vi "Is Close Delimiter.vi"(8 "Error In":errorcluster, 11 "Lexer In":refnum<class "Lexer.lvclass">) -> (0 "Error Out":errorcluster, 2 "Close Delimiter":bool, 3 "Lexer Out":refnum<class "Lexer.lvclass">)   [LabVIEW 2018, in "Toolkit.lvlib" / "Lexer.lvclass"]
uses:
  Lexer.lvclass
  Lexer.lvclass/Lexer.ctl
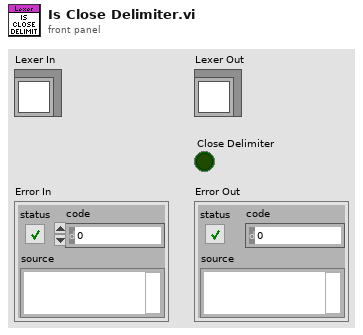
[diagram p1: front panel]
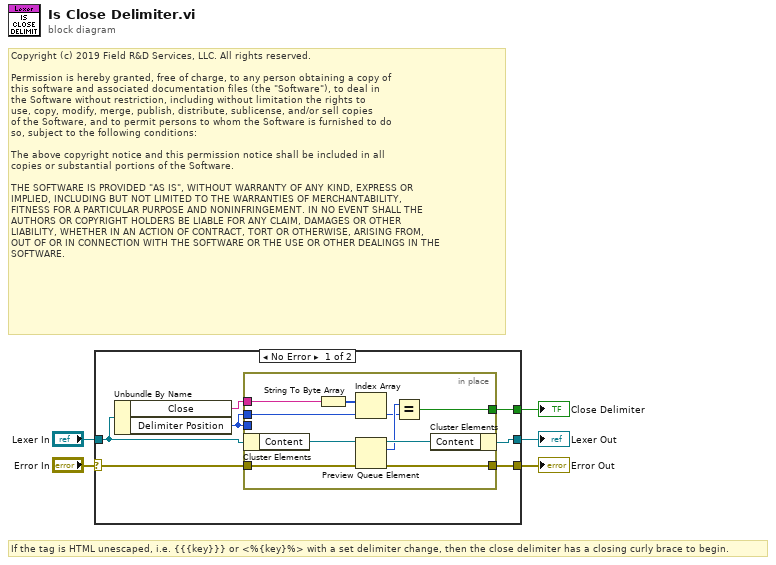
[diagram p0: block diagram]
diagram:
  # "Copyright (c) 2019 Field R&D Services, LLC. All rights reserved.\n\nPermission is hereby granted, free of charge, to any person obtaining a copy of\nthis software and associated documentation files (the \"Software\"), to deal in\nthe Software without restriction, including without limitation the rights to\nuse, copy, modify, merge, publish, distribute, sublicense, and/or sell copies\nof the Software, and to permit persons to whom the Software is furnished to do\nso, subject to the following conditions:\n\nThe above copyright notice and this permission notice shall be included in all\ncopies or substantial portions of the Software.\n\nTHE SOFTWARE IS PROVIDED \"AS IS\", WITHOUT WARRANTY OF ANY KIND, EXPRESS OR\nIMPLIED, INCLUDING BUT NOT LIMITED TO THE WARRANTIES OF MERCHANTABILITY,\nFITNESS FOR A PARTICULAR PURPOSE AND NONINFRINGEMENT. IN NO EVENT SHALL THE\nAUTHORS OR COPYRIGHT HOLDERS BE LIABLE FOR ANY CLAIM, DAMAGES OR OTHER\nLIABILITY, WHETHER IN AN ACTION OF CONTRACT, TORT OR OTHERWISE, ARISING FROM,\nOUT OF OR IN CONNECTION WITH THE SOFTWARE OR THE USE OR OTHER DEALINGS IN THE\nSOFTWARE."
  # "If the tag is HTML unescaped, i.e. {{{key}}} or <%{key}%> with a set delimiter change, then the close delimiter has a closing curly brace to begin."
  n1 = case shown="No Error" "Error In" {
    selector: "Error In" -> [w8 w24]
    tunnel: [w7 w24] -> w4
    tunnel: "Lexer In" -> [w12 w23]
    tunnel: [w11 w23] -> w2
    tunnel: [w9 _] -> w1
    frame No Error {
      n2 = Unbundle By Name(w12) -> ("Close"=w10:string, "Delimiter Position"=w6:i32)
      n3 = in-place {
        in-place-border: w6 -> [_]
        in-place-border: w10 -> [w22]
        in-place-border: [w17] -> w9
        in-place-border: w8 -> [w19]
        in-place-border: [w18] -> w7
        in-place-border: w6 -> [w15]
        n4 = in-place-cluster #1(w12) -> ("Content"=w21:refnum<queue>)
        n5 = String To Byte Array(string=w22) -> (unsigned byte array=w16:u8[])
        n6 = Index Array(array=w16, index=w15) -> (element=w13:u8)
        n7 = Preview Queue Element(queue=w21, error in (no error)=w19) -> (queue out=w20:refnum<queue>, element=w14:u8, error out=w18:errorcluster)  [unwired: 1 in, 1 out]
        n8 = Equal?(x=w14, y=w13) -> (x = y?=w17:bool)
        n9 = in-place-cluster #1("Content"=w20) -> (w11:refnum<class "Lexer.lvclass">)
      }
    }
    frame Error {
    }
  }
  "Error Out" <- w4
  "Lexer Out" <- w2
  "Close Delimiter" <- w1
